vi "Evaluate Operators.vi"(7 "Operators":T1) -> (8 "Operator":T2)   [LabVIEW 2025]
uses:
  Operator.ctl
  Operators.ctl
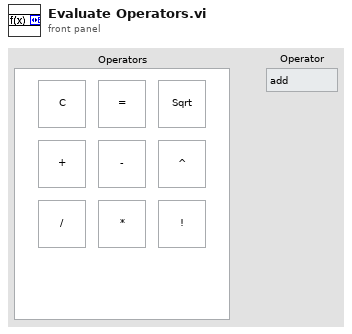
[diagram p1: front panel]
types:
  T1 = typedef "Operators.ctl" = cluster{"clear":bool, "equal":bool, "sqrt":bool, "add":bool, "sub":bool, "pwr":bool, "div":bool, "mul":bool, "fact":bool}
  T2 = typedef "Operator.ctl" = enum16{"add", "sub", "mul", "div", "pwr", "sqrt", "fact", "equal", "clear"}
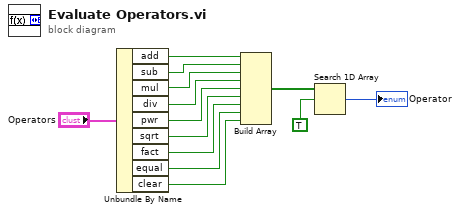
[diagram p0: block diagram]
diagram:
  n1 = Unbundle By Name("Operators") -> ("add"=w12:bool, "sub"=w11:bool, "mul"=w10:bool, "div"=w9:bool, "pwr"=w8:bool, "sqrt"=w7:bool, "fact"=w6:bool, "equal"=w5:bool, "clear"=w4:bool)
  n2 = Build Array(w12, w11, w10, w9, w8, w7, w6, w5, w4) -> (w3:bool[])
  n3 = Search 1D Array(1D array=w3, element=TRUE) -> (index of element=→"Operator":i32)  [unwired: 1 in]
